vi "openOutFile.vi"(8 "Entrée d'erreur":errorcluster caption="entrée d'erreur", 11 "Nom de l'analyse":string) -> (0 "Sortie d'erreur":errorcluster caption="sortie d'erreur", 3 "refnum en sortie":refnum<file>, 5 "chemin complet":path)   [LabVIEW 2019]
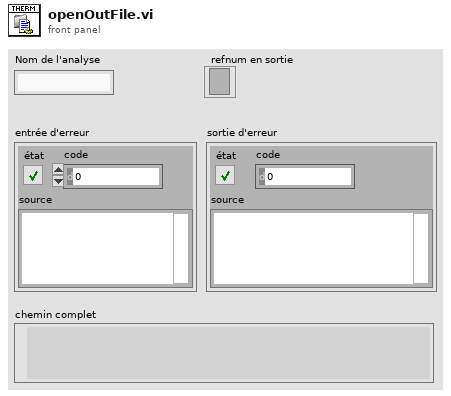
[diagram p1: front panel]
types:
  T1 = enum16{"open", "replace", "create", "open or create", "replace or create", "replace or create with confirmation"}
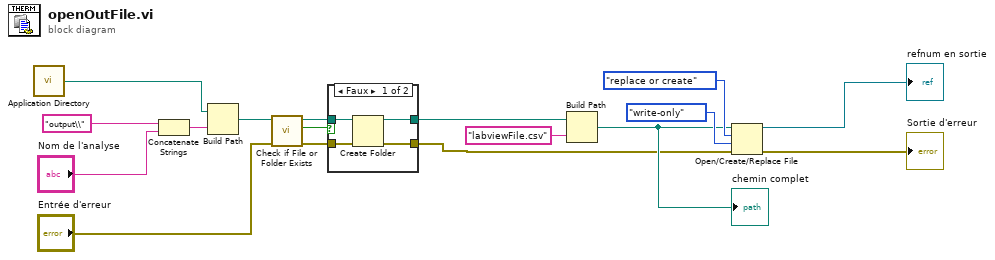
[diagram p0: block diagram]
diagram:
  n1 = call <vilib>:"Application Directory.vi"() -> ("Application Directory"=w11:path)
  n2 = Concatenate Strings("output\\" ("chaîne"), "Nom de l'analyse") -> (w12:string)
  n3 = Build Path(base path=w11, name or relative path=w12) -> (appended path=w4:path)
  n4 = call <vilib>:"Check if File or Folder Exists.vi"("error in (no error)"="Entrée d'erreur", "path"=w4) -> ("error out"=w1:errorcluster, "file or folder exists?"=w3:bool, "dup path"=w2:path)  [unwired: 7 in]
  n5 = case shown="Faux" w3 {
    tunnel: [w18 w23] -> w10
    tunnel: [w19 w22] -> w8
    tunnel: w2 -> [w21 w23]
    tunnel: w1 -> [w20 w22]
    frame False {
      n6 = Create Folder(path (use dialog)=w21, error in=w20) -> (created path=w18:path, error out=w19:errorcluster)  [unwired: 1 in, 1 out]
    }
    frame True {
    }
  }
  n7 = Build Path(base path=w10, name or relative path="labviewFile.csv" ("nom ou chemin relatif")) -> (appended path=w9:path)
  "chemin complet" <- w9
  n8 = Open/Create/Replace File(file path (use dialog)=w9, error in=w8, operation (0:open)=T1."replace or create" ("opération (0 : open)"), access (0:read/write)=enum16{"read/write", "read-only", "write-only"}."write-only" ("accès (0 : read/write)")) -> (refnum out=→"refnum en sortie":refnum<file>, error out=→"Sortie d'erreur":errorcluster)  [unwired: 2 in, 1 out]
